vi "Add2Plot.vi"(8 "error in":errorcluster, 10 "FP.Title":string="Add Yellow History to Plot", 11 "array":dbl[](array[numeric])=[0.5181035635992775, -3.2510837319166486, -1.0306751968313366, 0.3062937436986868, -2.240506246085896, -1.060295094536674, 2.517246942539657, -4.9894375599289775]) -> (0 "error out":errorcluster={"status"=TRUE, "code"=1, "source"="Enqueue Element in User Interface Global.vi->Add2Plot.vi"}, 3 "Cancelled?":bool)   [LabVIEW 2011]
doc: "Use this template to create a dialog box with event handling."
uses:
  Controls/Challenge.ctl
  Controls/Concentration Units.ctl
  Controls/Plot Parameters.ctl
  Controls/Data Analysis.ctl
  Controls/Data Processing.ctl
  Controls/User Interface Action.ctl
  Functional Global Data/Analysis Data.ctl
panel:
  in  "data analysis":T1={"analysis range"={1, 10}, "data processing"=enum."raw data"} {"analysis range" scale=1.0..5369.0}
  out "spectrum graph":dbl[](graph)
  in  "plot parameters":T3
  in  "challenge":T4
  in  "Cancel":bool
  in  "OK":bool
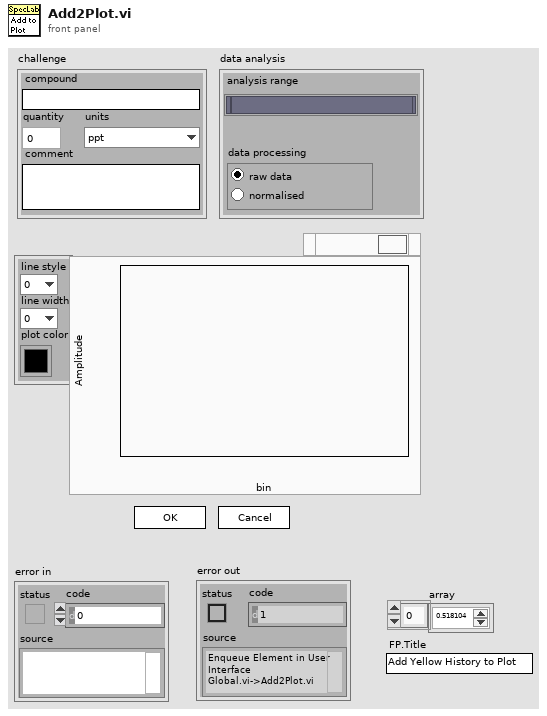
[diagram p1: front panel]
types:
  T1 = typedef "Data Analysis.ctl" = cluster{"analysis range":cluster{i32, i32}, "data processing":T2}
  T2 = typedef "Data Processing.ctl" = enum32{"raw data", "normalised"}
  T3 = typedef "Plot Parameters.ctl" = cluster{"line style":enum16{"0", "1", "2", "3", "4"}, "line width":enum16{"0", "1", "2", "3", "4", "5"}, "plot color":u32}
  T4 = typedef "Challenge.ctl" = cluster{"compound":string, "quantity":dbl, "units":T5, "comment":string}
  T5 = typedef "Concentration Units.ctl" = enum16{"ppt", "ppb", "ppm"}
  T6 = typedef "User Interface Action.ctl" = enum16{"Initialize", "Data Acquisition Disable", "Data View Disable", "Sample Set", "Sample Set 2D Data", "Sample Set x0 & dx", "Sample Add", "Sample Set Cursor", "Sample Set Offset & Multiplier", "Sample Set Axis Labels", "Sample Parameters Disabled", "Sample Parameters Update", "Run Update", "Run Set Offset & Multiplier", "Run Set Axis Labels", "Run Set Cursor", "Run Set Disabled", "Run Parameters Update", "Run Parameters Disabled", "Run Number Set", "Run Number Set Range", "Run Number Set Disabled", "Sample Number Set", "Sample Number Set Range", "Notes Set Value", "Update Plot", "Set Plot Parameters", "Update Concentration Plot", "Time Set", "Clear DAQ Display", "Clear Analysis Display", "Status Bar Set", "Progress Bar Set", "Display Mode Set", "Experiment Type Set", "Analysis Plot Average Set", "Stop"}
  T7 = typedef "Analysis Data.ctl" = enum16{"Initialize", "Add Plot", "Get Plots"}
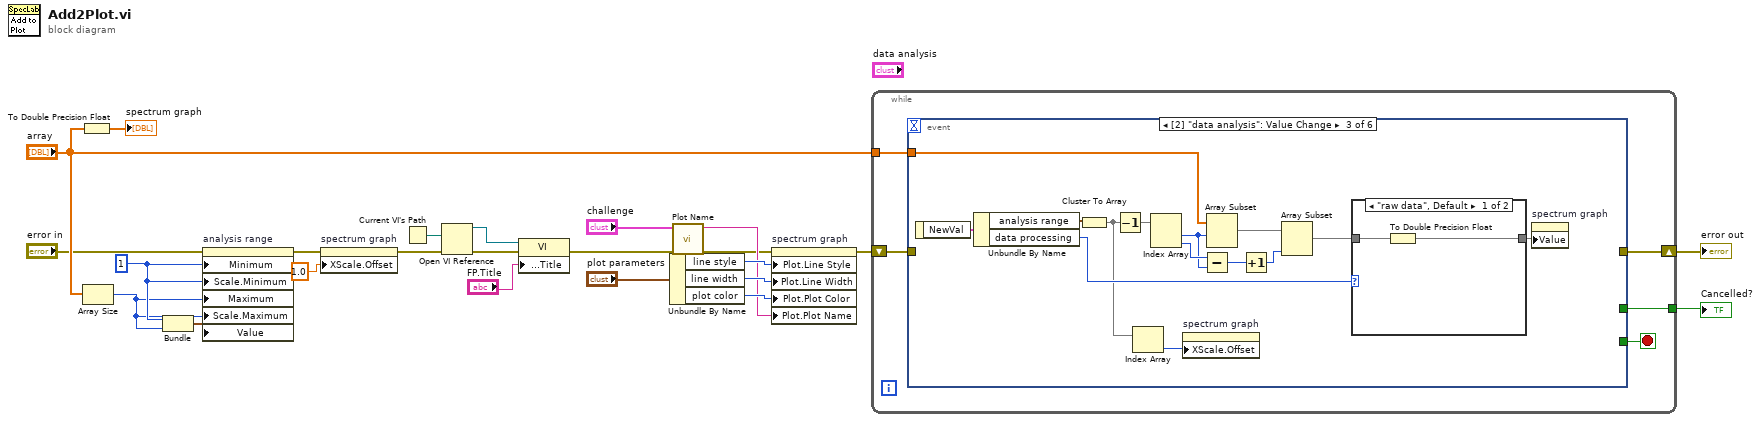
[diagram p0: block diagram]
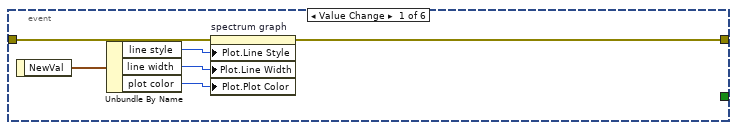
[diagram p2: hidden frame]
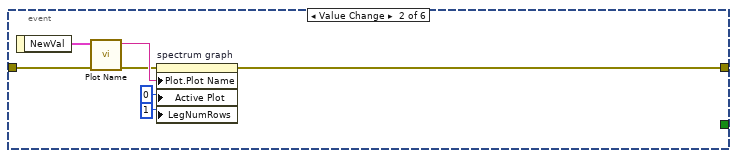
[diagram p3: hidden frame]
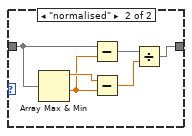
[diagram p4: hidden frame]
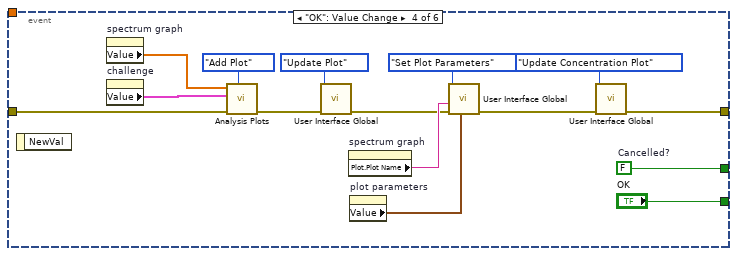
[diagram p5: hidden frame]
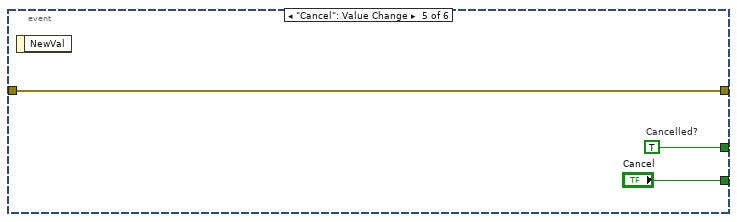
[diagram p6: hidden frame]
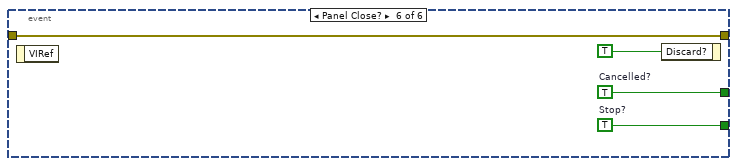
[diagram p7: hidden frame]
diagram:
  w3 = 1 ("Data Entry Limits:Minimum")
  n1 = To Double Precision Float(number="array") -> (double precision float=→"spectrum graph":dbl[])
  n2 = Array Size(array="array") -> (size(s)=w2:i32)
  n3 = Bundle("Data Entry Limits:Minimum"=w3, w2) -> (w1:cluster{"Data Entry Limits:Minimum":i32, i32})  [unwired: 1 in]
  n4 = property on="analysis range" class="Slide (strict)"(error in="error in", "Minimum"=w3, "Scale.Minimum"=w3, "Maximum"=w2, "Scale.Maximum"=w2, "Value"=w1) -> (error out=w5:errorcluster)  [unwired: 1 in, 1 out]
  n5 = property on="spectrum graph" class="WFGraph (strict)"(error in=w5, "XScale.Offset"=1.0 ("X Scale.Offset and Multiplier:Offset")) -> (error out=w4:errorcluster)  [unwired: 1 in, 1 out]
  n6 = Current VI's Path() -> (path=w12:path)
  n7 = Open VI Reference(vi path=w12, error in (no error)=w4) -> (vi reference=w13:refnum<vi>, error out=w10:errorcluster)  [unwired: 4 in]
  n8 = property class="VI"(reference=w13, error in=w10, "Front Panel.Title"="FP.Title") -> (error out=w8:errorcluster)  [unwired: 1 out]
  n9 = Unbundle By Name("plot parameters") -> ("line style"=w21:enum16{"0", "1", "2", "3", "4"}, "line width"=w20:enum16{"0", "1", "2", "3", "4", "5"}, "plot color"=w19:u32)
  n10 = call "Plot Name.vi"("error in"=w8, "challenge"="challenge") -> ("error out"=w16:errorcluster, "plot name"=w17:string)  [unwired: 7 in]
  n11 = property on="spectrum graph" class="WFGraph (strict)"(error in=w16, "Plot.Line Style"=w21, "Plot.Line Width"=w20, "Plot.Plot Color"=w19, "Plot.Plot Name"=w17) -> (error out=w15:errorcluster)  [unwired: 1 in, 1 out]
  n12 = while {
    tunnel: [w28] -> w24
    shift-right: [w26] -> w23
    shift-left: w15 -> [w27]
    tunnel: "array" -> [w25]
    stop <- w29 stop-if-true
    n13 = event shown="[2] \"data analysis\": Value Change" {
      selector: _ -> [_ _ _ _ _ _]
      dyn-events: _ -> [_ _ _ _ _ _]
      timeout: _ -> [_ _ _ _ _ _]
      tunnel: [_ _ _ "OK" "Cancel" w85] -> w29
      tunnel: [_ _ _ w79 w82 w84] -> w28
      tunnel: w27 -> [w31 w40 _ w76 w80 w83]
      tunnel: [w30 w36 _ w75 w80 w83] -> w26
      tunnel: w25 -> [_ _ w54 _ _ _]
      event Value Change {
        n14 = event-data() -> ("NewVal"=w35:T3)  [unwired: 1 in]
        n15 = Unbundle By Name(w35) -> ("line style"=w34:enum16{"0", "1", "2", "3", "4"}, "line width"=w33:enum16{"0", "1", "2", "3", "4", "5"}, "plot color"=w32:u32)
        n16 = property on="spectrum graph" class="WFGraph (strict)"(error in=w31, "Plot.Line Style"=w34, "Plot.Line Width"=w33, "Plot.Plot Color"=w32) -> (error out=w30:errorcluster)  [unwired: 1 in, 1 out]
      }
      event Value Change {
        n17 = event-data() -> ("NewVal"=w42:T4)  [unwired: 1 in]
        n18 = call "Plot Name.vi"("error in"=w40, "challenge"=w42) -> ("error out"=w37:errorcluster, "plot name"=w41:string)  [unwired: 7 in]
        n19 = property on="spectrum graph" class="WFGraph (strict)"(error in=w37, "Plot.Plot Name"=w41, "Active Plot"=u32 0, "LegNumRows"=u32 1 ("Active Plot")) -> (error out=w36:errorcluster)  [unwired: 1 in, 1 out]
      }
      event Value Change {
        n20 = event-data() -> ("NewVal"=w56:T1)  [unwired: 1 in]
        n21 = Unbundle By Name(w56) -> ("analysis range"=w55:cluster{i32, i32}, "data processing"=w52:T2)
        n22 = Cluster To Array(cluster=w55) -> (array=w46:i32[])
        n23 = Decrement(x=w46) -> (x-1=w48:i32[])
        n24 = Index Array(array=w46) -> (element=w45:i32)  [unwired: 1 in]
        n25 = Index Array(array=w48) -> (element #1=w47:i32, element #2=w51:i32)  [unwired: 2 in]
        n26 = property on="spectrum graph" class="WFGraph (strict)"("XScale.Offset"=w45) -> ()  [unwired: 2 in, 2 out]
        n27 = Subtract(x=w51, y=w47) -> (x-y=w44:i32)
        n28 = Array Subset(array=w54, index=w47) -> (w53:dbl[])  [unwired: 1 in]
        n29 = Increment(x=w44) -> (x+1=w43:i32)
        n30 = Array Subset(array=w53, length=w43) -> (w50:dbl[])  [unwired: 1 in]
        n31 = case shown="\"raw data\", Default" w52 {
          tunnel: w50 -> [w58 w64]
          tunnel: [w57 w59] -> w49
          frame "raw data", Default {
            n32 = To Double Precision Float(number=w58) -> (double precision float=w57:dbl[])
          }
          frame "normalised" {
            n33 = Array Max & Min(array=w64) -> (max value=w63:dbl, min value=w62:dbl)  [unwired: 2 out]
            n34 = Subtract(x=w64, y=w62) -> (x-y=w60:dbl[])
            n35 = Subtract(x=w63, y=w62) -> (x-y=w61:dbl)
            n36 = Divide(x=w60, y=w61) -> (x/y=w59:dbl[])
          }
        }
        n37 = property on="spectrum graph" class="WFGraph (strict)"("Value"=w49) -> ()  [unwired: 2 in, 2 out]
      }
      event "OK": Value Change {
        w79 = FALSE  # Cancelled?
        n38 = event-data() -> ()  [unwired: 1 in, 1 out]
        n39 = property on="spectrum graph" class="WFGraph (strict)"() -> ("Value"=w65:dbl[])  [unwired: 2 in, 2 out]
        n40 = property on="challenge" class="Clust (strict)"() -> ("Value"=w77:T4)  [unwired: 2 in, 2 out]
        n41 = call "Analysis Plots.vi"("action"=Analysis_Data."Add Plot" ("Action"), "error in"=w76, "challenge"=w77, "IMS spectrum"=w65) -> ("error out"=w68:errorcluster)  [unwired: 5 in, 2 out]
        n42 = call "User Interface Global.vi"("error in"=w68, "action"=User_Interface_Action."Update Plot" ("Action")) -> ("error out"=w66:errorcluster)  [unwired: 9 in]
        n43 = property on="spectrum graph" class="WFGraph (strict)"() -> ("Plot.Plot Name"=w74:string)  [unwired: 2 in, 2 out]
        n44 = property on="plot parameters" class="Clust (strict)"() -> ("Value"=w73:T3)  [unwired: 2 in, 2 out]
        n45 = call "User Interface Global.vi"("data2"=w73, "error in"=w66, "data1"=w74, "action"=User_Interface_Action."Set Plot Parameters" ("Action")) -> ("error out"=w67:errorcluster)  [unwired: 7 in]
        n46 = call "User Interface Global.vi"("error in"=w67, "action"=User_Interface_Action."Update Concentration Plot" ("Action")) -> ("error out"=w75:errorcluster)  [unwired: 9 in]
      }
      event "Cancel": Value Change {
        w82 = TRUE  # Cancelled?
        n47 = event-data() -> ()  [unwired: 1 in, 1 out]
      }
      event Panel Close? {
        w84 = TRUE  # Cancelled?
        w85 = TRUE  # Stop?
        n48 = event-data() -> ()  [unwired: 1 in, 1 out]
        n49 = event-data("Discard?"=TRUE) -> ()  [unwired: 1 in, 1 out]
      }
    }
  }
  "Cancelled?" <- w24
  "error out" <- w23
